vi "Generate Parameter.vi"(8 "error in (no error)":errorcluster, 10 "Variant data":variant, 11 "Type Enum":T1) -> (0 "error out":errorcluster, 3 "parameter information":T4)   [LabVIEW 2011]
uses:
  <vilib>/addons/database/Auxilliary.llb/DB Tools DataTypes.ctl
  <vilib>/addons/database/Auxilliary.llb/DB Tools Parameter Dir.ctl
  <vilib>/Utility/VariantDataType/Type.ctl
  <vilib>/addons/database/Auxilliary.llb/DB Tools Parameter Info.ctl
  <vilib>/addons/database/NI_Database_API.lvlib
  <vilib>/Utility/VariantDataType/VariantType.lvlib
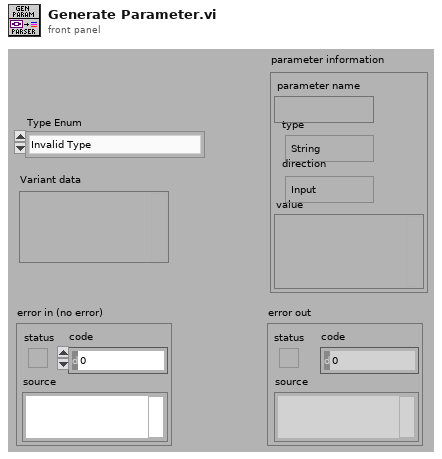
[diagram p1: front panel]
types:
  T1 = typedef "VariantType.lvlib/Type.ctl" = enum8{"Invalid Type", "Void", "I8", "I16", "I32", "I64", "U8", "U16", "U32", "U64", "Single Float", "Double Float", "Extended Float", "Single Complex", "Double Complex", "Extended Complex", "Enum U8", "Enum U16", "Enum U32", "Enum U64", "Single Float With Unit", "Double Float With Unit", "Extended Float With Unit", "Single Complex with Unit", "Double Complex with Unit", "Extended Complex with Unit", "Boolean", "String", "Path", "Picture", "Tag", "Array", "Cluster", "Variant", "LV Variant", "Waveform", "Timestamp", "Digital Waveform", "Digital Data", "ExpressData", "Refnum", "External Data", "VI", "Poly VI", "LabVIEW Class Instance", "Fixed Point"}
  T2 = typedef "NI_Database_API.lvlib/DB Tools DataTypes.ctl" = enum16{"String", "Long (I32)", "Single (SGL)", "Double (DBL)", "Date/Time", "Binary"}
  T3 = typedef "NI_Database_API.lvlib/DB Tools Parameter Dir.ctl" = enum32{"Input", "Output", "Input/Output", "Return Value"}
  T4 = cluster{"parameter name":string, "type":T2, "direction":T3, "value":variant}
  T5 = typedef "NI_Database_API.lvlib/DB Tools Parameter Info.ctl" = cluster{"parameter name":string, "type":T2, "direction":T3, "value":variant}
  T6 = typedef "LVDateTimeRec.ctl" = cluster{"fractional second":dbl, "second":i32, "minute":i32, "hour":i32, "day of month":i32, "month":i32, "year":i32, "day of week":i32, "day of year":i32, "DST":i32}
  T7 = typedef "VariantType.lvlib/RefnumType.ctl" = enum16{"NotARefnum", "UnknownRefnum", "Generic", "Datalog", "ByteStream", "Device", "Occurence", "TCPNetConnection", "Auto", "Menu", "Imaq", "Hardware", "DataSocket", "Visa", "IVI", "UDPNetConnection", "Notifier", "Queue", "Irda", "EventReg", "DotNet", "UserEvent", "Callback", "UNUSED_EMPTY_POSITION", "BlueToothNetConnection", "LVObjApp", "LVObjVI", "LVObjUnknown", "GenericClass", "UserDefinedRefnumTag", "DataValue"}
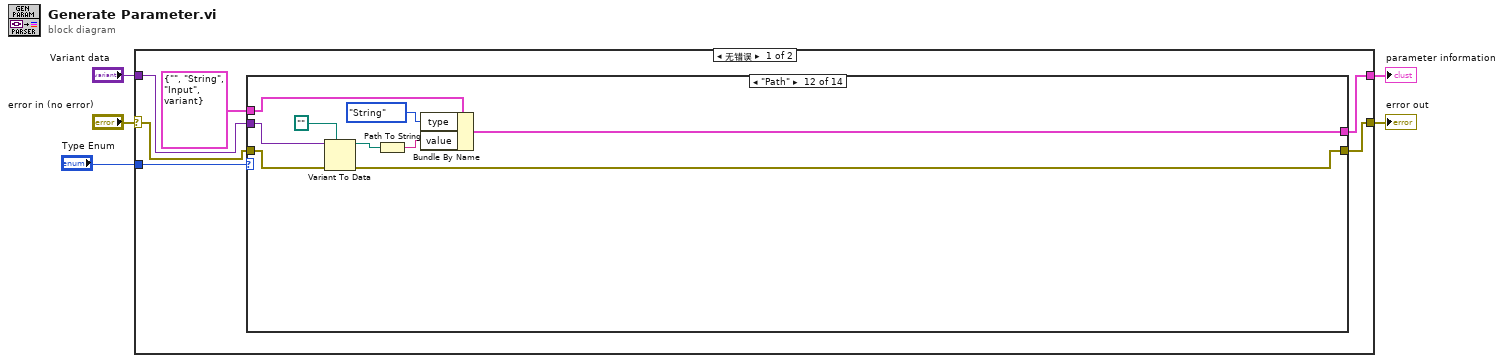
[diagram p0: block diagram]
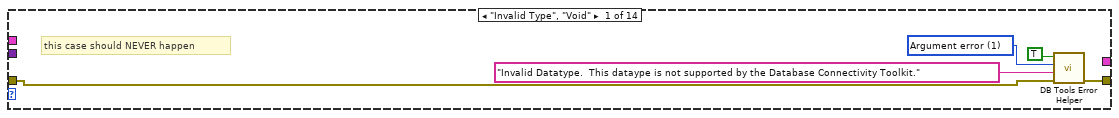
[diagram p2: hidden frame]
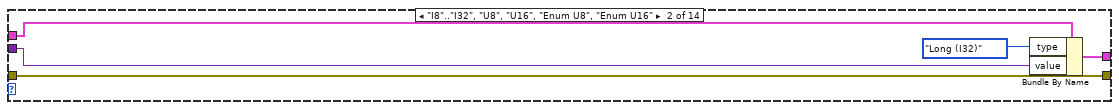
[diagram p3: hidden frame]
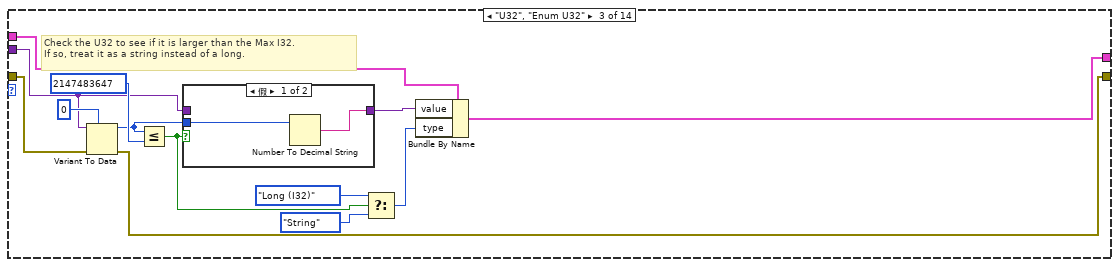
[diagram p4: hidden frame]
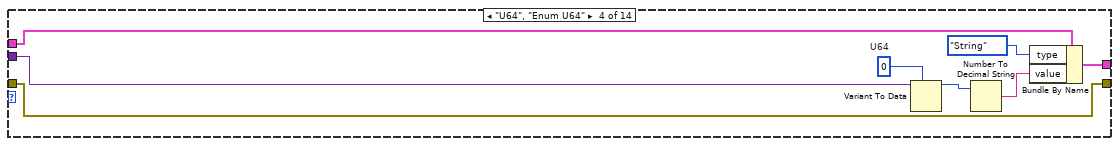
[diagram p6: hidden frame]
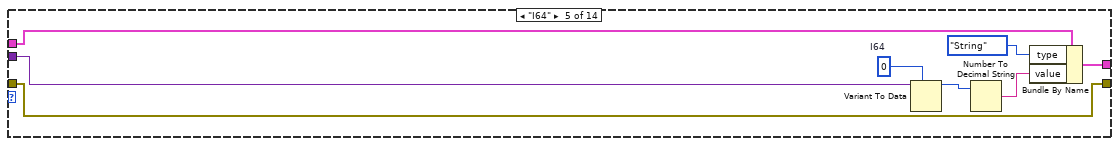
[diagram p7: hidden frame]
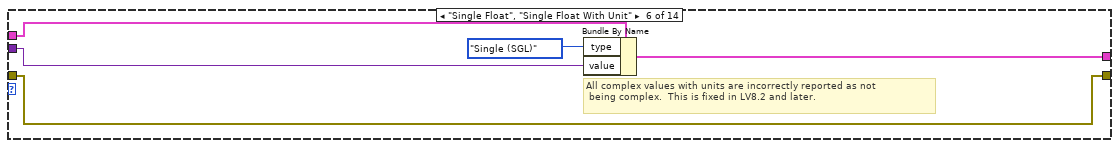
[diagram p8: hidden frame]
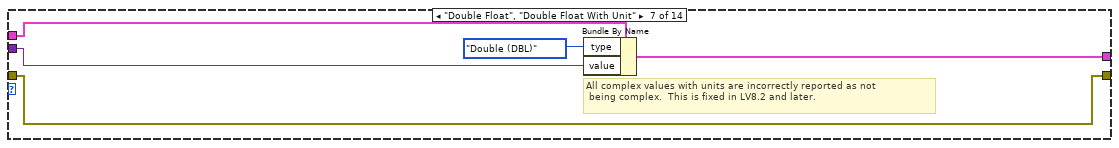
[diagram p9: hidden frame]
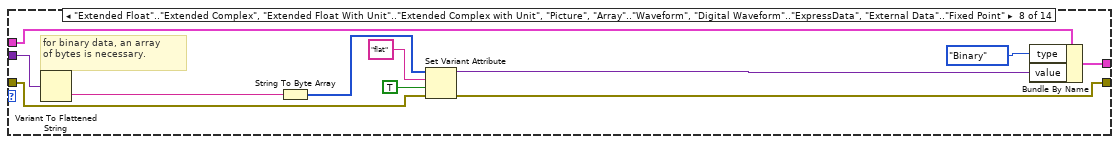
[diagram p10: hidden frame]
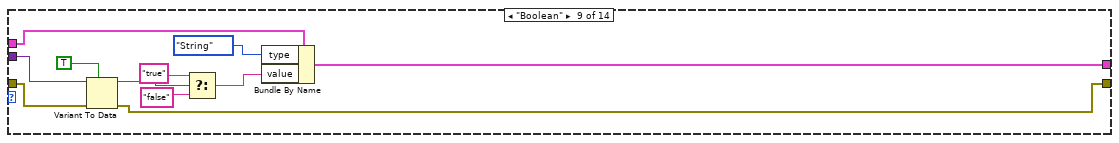
[diagram p11: hidden frame]
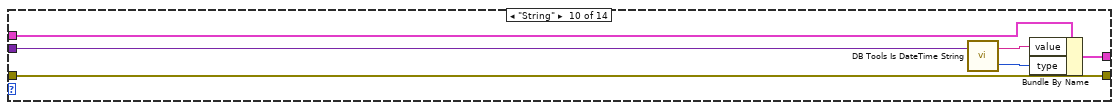
[diagram p12: hidden frame]
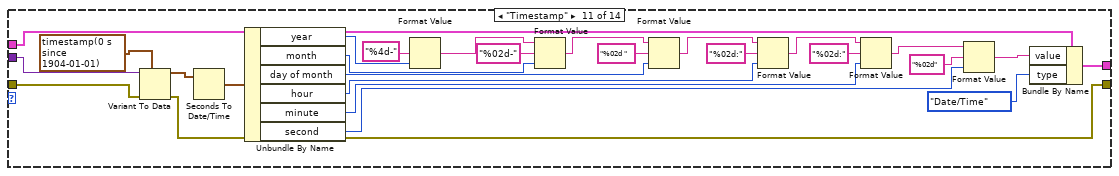
[diagram p13: hidden frame]
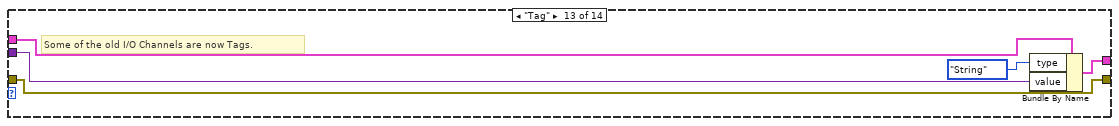
[diagram p14: hidden frame]
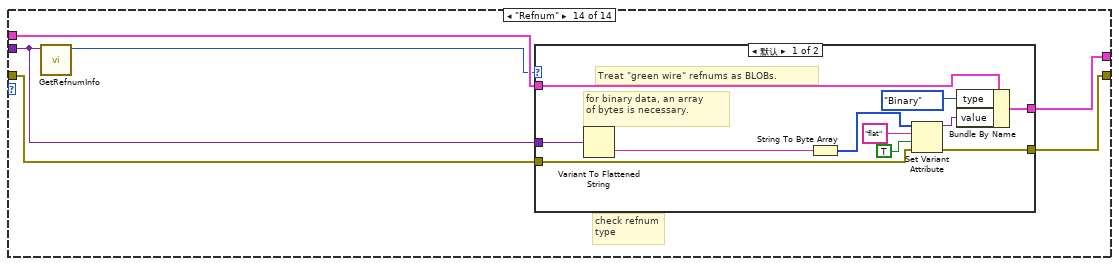
[diagram p15: hidden frame]
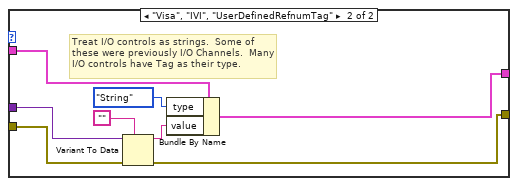
[diagram p16: hidden frame]
diagram:
  n1 = case shown="无错误" "error in (no error)" {
    selector: "error in (no error)" -> [w6 w158]
    tunnel: [w10 _] -> w2
    tunnel: "Variant data" -> [w9 _]
    tunnel: "Type Enum" -> [w8 _]
    tunnel: [w7 w158] -> w4
    frame No Error {
      n2 = case shown="\"Path\"" w8 {
        tunnel: [w13 w17 w27 w43 w51 w55 w60 w64 w76 w87 w115 w119 w129 w136] -> w7
        tunnel: T5 {"parameter name"="", "type"=enum."String", "direction"=enum."Input", "value"=variant} ("Parameter Cluster") -> [_ w21 w34 w45 w53 w57 w62 w73 w80 w89 w118 w123 w131 w138]
        tunnel: w6 -> [w12 w17 w28 w43 w51 w55 w60 w65 w77 w87 w116 w120 w129 w137]
        tunnel: w9 -> [_ w20 w24 w41 w49 w56 w61 w67 w82 w91 w117 w127 w130 w135]
        tunnel: [_ w18 w29 w42 w50 w54 w59 w66 w78 w86 w92 w121 w128 w133] -> w10
        frame "Invalid Type", "Void" {
          w15 = 1 items=["No error", "Argument error", "Memory is full", "Out of zone", "End of file", "File already open", "Generic file I/O error", "File not found", "File permission error", "Disk is full", "Duplicate path", "Too many files open", "System feature not enabled", "Resource file not found", "Cannot add resource", "Resource not found", "Image not found", "Image memory error", "Pen does not exist", "Config type invalid", "Config token not found", "Config parse error", "Config memory error", "Bad external code format", "Bad external code offset", "External code not present", "Null window", "Destroy window error", "Null menu", "Print aborted", "Bad print record", "Print driver error", "Windows error during printing", "Memory error during printing", "Print dialog error", "Generic print error", "Invalid device refnum", "Device not found", "Device parameter error", "Device unit error", "Cannot open device", "Device call aborted", "Generic error", "Cancelled by user", "Object ID too low", "Object ID too high", "Object not in heap", "Unknown heap", "Unknown object (invalid DefProc)", "Unknown object (DefProc not in table)", "Message out of range", "Invalid (null) method", "Unknown message", "Manager call not supported", "Bad address", "Network operation in progress", "Network operation timed out", "Connection is busy", "Network attribute not supported", "Network error", "Address in use", "System out of memory", "Connection aborted", "Connection refused", "Not connected", "Already connected", "Connection closed", "Initialization error (interapplication manager)", "Bad occurrence", "Wait on unbound occurrence handler", "Occurrence queue overflow", "Datalog type conflict", "Unused", "Unrecognized type (interapplication manager)", "Memory corrupt", "Failed to make temporary DLL", "Old CIN version", "Drag socket not found", "Failed to load drop-object", "Failed to register OLE object", "Failed to release OLE object", "Format specifier type mismatch", "Unknown format specifier", "Too few format specifiers", "Too many format specifiers", "Scan failed", "Newer CIN version", "Error converting to variant", "Runtime menu error", "Password tampered", "Variant attribute not found", "Incompatible variant data type", "Event data is not available", "Event Store is not present", "Occurrence is not found", "Event Queue is not created", "Event info is not available", "Refnum passed is NULL", "Error retrieving Class GUID", "Error retrieving CoClass GUID", "Error retrieving TypeLib GUID.", ""]
          # "this case should NEVER happen"
          n3 = call <vilib>:"DB Tools Error Helper.vi"("Overriding error or warning"=w12, "source"="Invalid Datatype.  This dataype is not supported by the Database Connectivity Toolkit.", "code"=w15, "status"=TRUE) -> ("error out"=w13:errorcluster)  [unwired: 7 out]
        }
        frame "I8".."I32", "U8", "U16", "Enum U8", "Enum U16" {
          n4 = Bundle By Name(cluster=w21, "type"=DB_Tools_DataTypes."Long (I32)", "value"=w20) -> (w18:T5)
        }
        frame "U32", "Enum U32" {
          # "Check the U32 to see if it is larger than the Max I32.  \nIf so, treat it as a string instead of a long."
          n5 = Variant To Data(error in=w28, type=u32 0, Variant=w24) -> (data=w23:u32, error out=w27:errorcluster)
          n6 = Less Or Equal?(x=w23, y=2147483647) -> (x <= y?=w25:bool)
          n7 = case shown="假" w25 {
            tunnel: w24 -> [_ w37]
            tunnel: w23 -> [w36 _]
            tunnel: [w35 w37] -> w22
            frame False {
              n8 = Number To Decimal String(number=w36) -> (decimal integer string=w35:string)  [unwired: 1 out]
            }
            frame True {
            }
          }
          n9 = Select(t=DB_Tools_DataTypes."Long (I32)" ("type"), s=w25, f=DB_Tools_DataTypes."String" ("type")) -> (s? t:f=w26:T2)
          n10 = Bundle By Name(cluster=w34, "value"=w22, "type"=w26) -> (w29:T5)
        }
        frame "U64", "Enum U64" {
          w38 = u64 0  # U64
          n11 = Variant To Data(type=w38, Variant=w41) -> (data=w40:u64)  [unwired: 1 in, 1 out]
          n12 = Number To Decimal String(number=w40) -> (decimal integer string=w39:string)  [unwired: 1 out]
          n13 = Bundle By Name(cluster=w45, "type"=DB_Tools_DataTypes."String", "value"=w39) -> (w42:T5)
        }
        frame "I64" {
          w46 = i64 0  # I64
          n14 = Variant To Data(type=w46, Variant=w49) -> (data=w48:i64)  [unwired: 1 in, 1 out]
          n15 = Number To Decimal String(number=w48) -> (decimal integer string=w47:string)  [unwired: 1 out]
          n16 = Bundle By Name(cluster=w53, "type"=DB_Tools_DataTypes."String", "value"=w47) -> (w50:T5)
        }
        frame "Single Float", "Single Float With Unit" {
          # "All complex values with units are incorrectly reported as not\n being complex.  This is fixed in LV8.2 and later."
          n17 = Bundle By Name(cluster=w57, "type"=DB_Tools_DataTypes."Single (SGL)", "value"=w56) -> (w54:T5)
        }
        frame "Double Float", "Double Float With Unit" {
          # "All complex values with units are incorrectly reported as not\n being complex.  This is fixed in LV8.2 and later."
          n18 = Bundle By Name(cluster=w62, "type"=DB_Tools_DataTypes."Double (DBL)", "value"=w61) -> (w59:T5)
        }
        frame "Extended Float".."Extended Complex", "Extended Float With Unit".."Extended Complex with Unit", "Picture", "Array".."Waveform", "Digital Waveform".."ExpressData", "External Data".."Fixed Point" {
          # "for binary data, an array\nof bytes is necessary."
          n19 = Variant To Flattened String(Variant=w67) -> (data string=w72:string)  [unwired: 1 out]
          n20 = String To Byte Array(string=w72) -> (unsigned byte array=w69:u8[])
          n21 = Set Variant Attribute(Variant=w69, name="flat", value=TRUE, error in=w65) -> (Variant out=w68:variant, error out=w64:errorcluster)  [unwired: 1 out]
          n22 = Bundle By Name(cluster=w73, "type"=DB_Tools_DataTypes."Binary", "value"=w68) -> (w66:T5)
        }
        frame "Boolean" {
          n23 = Variant To Data(error in=w77, type=TRUE ("Boolean"), Variant=w82) -> (data=w75:bool, error out=w76:errorcluster)
          n24 = Select(t="true", s=w75, f="false") -> (s? t:f=w79:string)
          n25 = Bundle By Name(cluster=w80, "type"=DB_Tools_DataTypes."String", "value"=w79) -> (w78:T5)
        }
        frame "String" {
          n26 = call <vilib>:"DB Tools Is DateTime String.vi"("string or date/time"=w91) -> ("database data type"=w88:T2, "data"=w90:string)  [unwired: 1 out]
          n27 = Bundle By Name(cluster=w89, "value"=w90, "type"=w88) -> (w86:T5)
        }
        frame "Timestamp" {
          n28 = Variant To Data(error in=w116, type=timestamp(0 s since 1904-01-01), Variant=w117) -> (data=w113:timestamp, error out=w115:errorcluster)
          n29 = Seconds To Date/Time(time stamp (now)=w113) -> (date time rec=w103:T6)  [unwired: 1 out]
          n30 = Unbundle By Name(w103) -> ("year"=w109:i32, "month"=w110:i32, "day of month"=w100:i32, "hour"=w102:i32, "minute"=w101:i32, "second"=w104:i32)
          n31 = Format Value(format string="%4d-", value (0)=w109) -> (output string=w93:string)  [unwired: 1 out]
          n32 = Format Value(string ("")=w93, format string="%02d-", value (0)=w110) -> (output string=w94:string)
          n33 = Format Value(string ("")=w94, format string="%02d ", value (0)=w100) -> (output string=w95:string)
          n34 = Format Value(string ("")=w95, format string="%02d:", value (0)=w102) -> (output string=w96:string)
          n35 = Format Value(string ("")=w96, format string="%02d:", value (0)=w101) -> (output string=w97:string)
          n36 = Format Value(string ("")=w97, format string="%02d", value (0)=w104) -> (output string=w98:string)
          n37 = Bundle By Name(cluster=w118, "value"=w98, "type"=DB_Tools_DataTypes."Date/Time" ("database data type")) -> (w92:T5)
        }
        frame "Path" {
          n38 = Variant To Data(error in=w120, type=path "", Variant=w127) -> (data=w125:path, error out=w119:errorcluster)
          n39 = Path To String(path=w125) -> (string=w122:string)
          n40 = Bundle By Name(cluster=w123, "type"=DB_Tools_DataTypes."String", "value"=w122) -> (w121:T5)
        }
        frame "Tag" {
          # "Some of the old I/O Channels are now Tags."
          n41 = Bundle By Name(cluster=w131, "type"=DB_Tools_DataTypes."String", "value"=w130) -> (w128:T5)
        }
        frame "Refnum" {
          # "check refnum type"
          n42 = call <vilib>:"GetRefnumInfo.vi"("Variant"=w135) -> ("ReferenceType"=w134:T7)  [unwired: 1 in, 9 out]
          n43 = case shown="默认" w134 {
            tunnel: w138 -> [w143 w156]
            tunnel: w137 -> [w141 w153]
            tunnel: [w140 w152] -> w136
            tunnel: w135 -> [w142 w151]
            tunnel: [w139 w150] -> w133
            frame Default {
              # "Treat \"green wire\" refnums as BLOBs."
              # "for binary data, an array\nof bytes is necessary."
              n44 = Variant To Flattened String(Variant=w142) -> (data string=w148:string)  [unwired: 1 out]
              n45 = String To Byte Array(string=w148) -> (unsigned byte array=w145:u8[])
              n46 = Set Variant Attribute(Variant=w145, name="flat", value=TRUE, error in=w141) -> (Variant out=w144:variant, error out=w140:errorcluster)  [unwired: 1 out]
              n47 = Bundle By Name(cluster=w143, "type"=DB_Tools_DataTypes."Binary", "value"=w144) -> (w139:T5)
            }
            frame "Visa", "IVI", "UserDefinedRefnumTag" {
              # "Treat I/O controls as strings.  Some of these were previously I/O Channels.  Many I/O controls have Tag as their type."
              n48 = Variant To Data(error in=w153, type="", Variant=w151) -> (data=w155:string, error out=w152:errorcluster)
              n49 = Bundle By Name(cluster=w156, "type"=DB_Tools_DataTypes."String", "value"=w155) -> (w150:T5)
            }
          }
        }
      }
    }
    frame Error {
    }
  }
  "parameter information" <- w2
  "error out" <- w4
